vi "I2C Communication.vi"(8 "error in":errorcluster) -> ()   [LabVIEW 2014]
uses:
  <vilib>/Rock Robotics/WPI/DriverStation/WPI_DriverStationRobotMode2.ctl
  <vilib>/Rock Robotics/WPI/DriverStation/WPI_DriverStationAllianceInfo.ctl
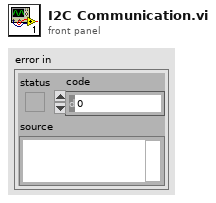
[diagram p1: front panel]
types:
  T1 = typedef "WPI_DriverStationRobotMode2.ctl" = enum16{"Autonomous Disabled", "Autonomous Enabled", "Teleop Disabled", "Teleop Enabled", "Disconnected", "Finish", "Test Disabled", "Test Enabled", "Emergency Stopped"}
  T2 = typedef "WPI_DriverStationAllianceInfo.ctl" = enum16{"Red", "Blue", "Invalid"}
  T3 = typedef "WPI_I2CDevRef.ctl" = cluster{"DevStatus":errorcluster, "Controller":T4, "Device Address":u8, "Handle":i32, "I2C Bus":T5}
  T4 = typedef "FPGA_TypedefDigitalModule.ctl" = enum16{"Controller 1"}
  T5 = typedef "i2c_bus.ctl" = enum16{"I2C On-Board", "I2C MXP", "Invalid"}
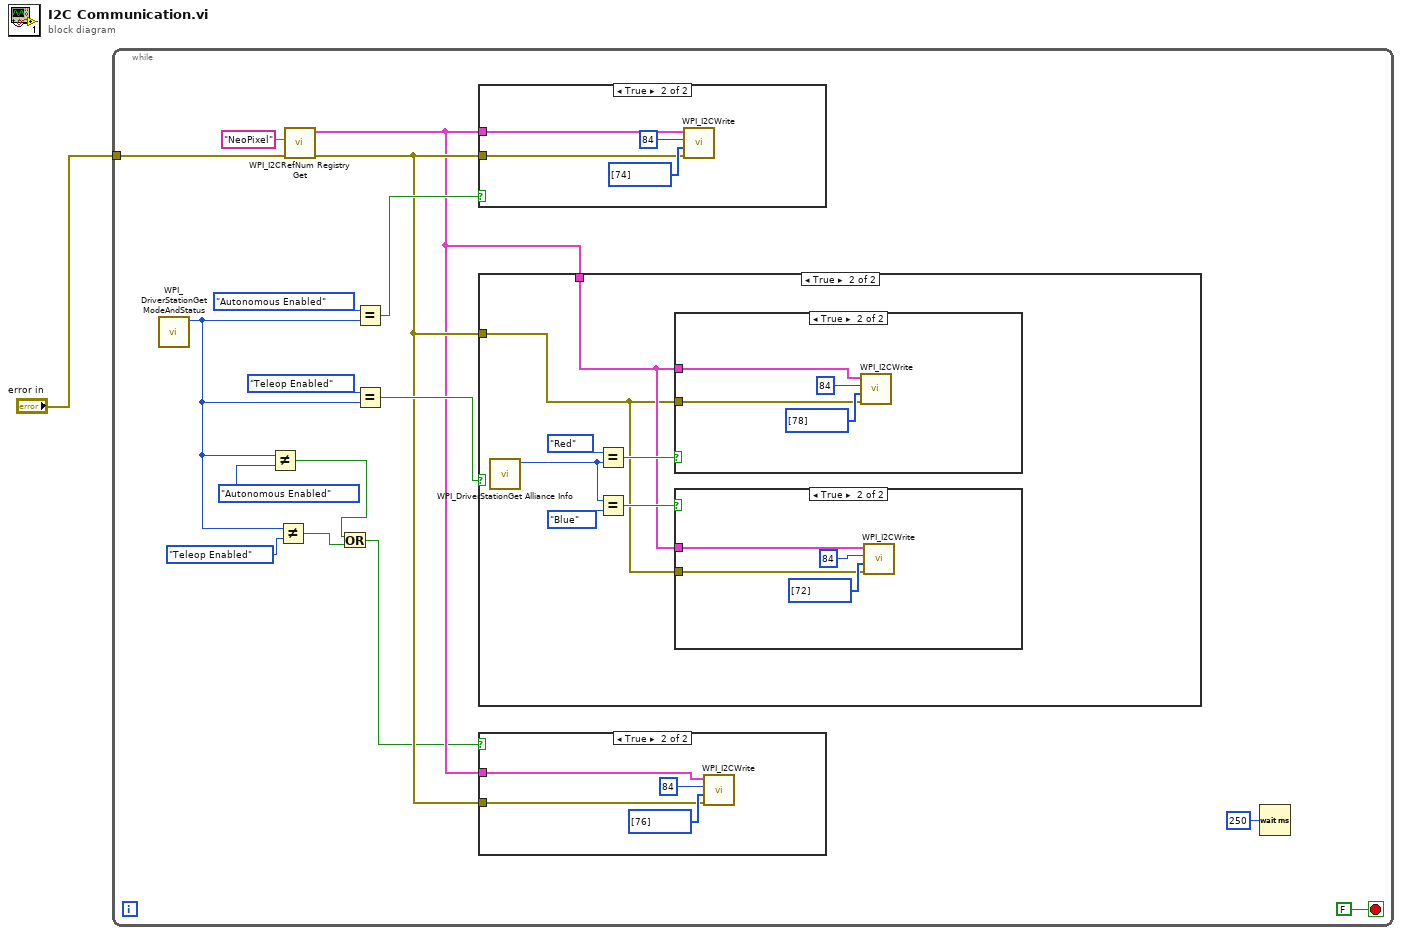
[diagram p0: block diagram]
diagram:
  n1 = while {
    tunnel: "error in" -> [w11]
    stop <- FALSE stop-if-true
    n2 = call <vilib>:"WPI_DriverStationGetModeAndStatus.vi"() -> ("Robot Mode"=w6:T1)  [unwired: 10 in, 1 out]
    n3 = Not Equal?(x=w6, y=WPI_DriverStationRobotMode2."Autonomous Enabled") -> (x != y?=w4:bool)
    n4 = Not Equal?(x=w6, y=WPI_DriverStationRobotMode2."Teleop Enabled") -> (x != y?=w3:bool)
    n5 = call <vilib>:"WPI_I2CRefNum Registry Get.vi"("error in (no error)"=w11, "refnum name"="NeoPixel") -> ("error out"=w9:errorcluster, "I2CDevRef"=w8:T3)  [unwired: 8 in]
    n6 = Or(x=w4, y=w3) -> (x .or. y?=w2:bool)
    n7 = Equal?(x=WPI_DriverStationRobotMode2."Autonomous Enabled" ("Robot Mode"), y=w6) -> (x = y?=w14:bool)
    n8 = Equal?(x=WPI_DriverStationRobotMode2."Teleop Enabled" ("Robot Mode"), y=w6) -> (x = y?=w15:bool)
    n9 = case shown="True" w14 {
      tunnel: w8 -> [_ w38]
      tunnel: w9 -> [_ w37]
      frame False {
      }
      frame True {
        n10 = call <vilib>:"WPI_I2CWrite.vi"("error in (no error)"=w37, "I2CDataToSend"=u8[] [74], "I2CRegister"=u8 84, "I2CDevRef"=w38) -> ()  [unwired: 6 in, 2 out]
      }
    }
    n11 = case shown="True" w15 {
      tunnel: w8 -> [_ w23]
      tunnel: w9 -> [_ w22]
      frame False {
      }
      frame True {
        n12 = call <vilib>:"WPI_DriverStationGet Alliance Info.vi"() -> ("Alliance"=w27:T2)  [unwired: 10 in, 1 out]
        n13 = Equal?(x=WPI_DriverStationAllianceInfo."Red" ("Alliance"), y=w27) -> (x = y?=w25:bool)
        n14 = Equal?(x=w27, y=WPI_DriverStationAllianceInfo."Blue") -> (x = y?=w24:bool)
        n15 = case shown="True" w25 {
          tunnel: w23 -> [_ w34]
          tunnel: w22 -> [_ w33]
          frame False {
          }
          frame True {
            n16 = call <vilib>:"WPI_I2CWrite.vi"("error in (no error)"=w33, "I2CDataToSend"=u8[] [78], "I2CRegister"=u8 84, "I2CDevRef"=w34) -> ()  [unwired: 6 in, 2 out]
          }
        }
        n17 = case shown="True" w24 {
          tunnel: w23 -> [_ w30]
          tunnel: w22 -> [_ w29]
          frame False {
          }
          frame True {
            n18 = call <vilib>:"WPI_I2CWrite.vi"("error in (no error)"=w29, "I2CDataToSend"=u8[] [72], "I2CRegister"=u8 84, "I2CDevRef"=w30) -> ()  [unwired: 6 in, 2 out]
          }
        }
      }
    }
    n19 = case shown="True" w2 {
      tunnel: w9 -> [_ w19]
      tunnel: w8 -> [_ w18]
      frame False {
      }
      frame True {
        n20 = call <vilib>:"WPI_I2CWrite.vi"("error in (no error)"=w19, "I2CDataToSend"=u8[] [76], "I2CRegister"=u8 84, "I2CDevRef"=w18) -> ()  [unwired: 6 in, 2 out]
      }
    }
    n21 = Wait (ms)(milliseconds to wait=u32 250) -> ()  [unwired: 1 out]
  }
